vi "sensor wrapper rob.vi"(6 "Degrees":dbl, 8 "error in (no error)":errorcluster, 9 "sensor y":fxp<+/-,64,32>, 10 "Sensor x":fxp<+/-,64,32>, 11 "map reference in":refnum<data-value>) -> (0 "error out":errorcluster, 3 "map reference out 2":refnum<data-value>)   [LabVIEW 2012]
uses:
  <vilib>/rvi/interface/nirviOpenFPGA/nirviOpenFPGA.xnode
  <vilib>/rvi/interface/nirviCloseFPGA/nirviCloseFPGA.xnode
  <vilib>/FPGAPlugInAG/Dynamic/niLvFpga_Close_Dynamic.vi
  <vilib>/rvi/interface/nirviReadWriteControl/nirviReadWriteControl.xnode
  NiFpgaLv.dll
  <vilib>/Utility/error.llb/Error Cluster From Error Code.vi
  <vilib>/rvi/interface/Simulation/niFpgaSimulationCallBeginRW.vi
  <vilib>/rvi/errors/niLvFpgaAdjustHostInterfaceError.vi
  <vilib>/robotics/Navigation/shared/WorldMap/OccupancyGridWorldMap/NI_Robotics_OccupancyGridWorldMap.lvclass
  fpgatrig.vi
  <vilib>/rvi/interface/RandomDataEmulation/nirviRandomDataOpen.vi
  <vilib>/rvi/interface/common/niFpgaCacheSessionInfoDynamic.vi
panel:
  in  "distance":fxp<+/-,64,32>
  out "Rounded y":fxp<+/-,64,32>
  out "Rounded x":fxp<+/-,64,32>
  out "Detected x":fxp<+/-,64,32>
  out "Detected y":fxp<+/-,64,32>
  # "Add into own loop so it updates map independent of disicion making"
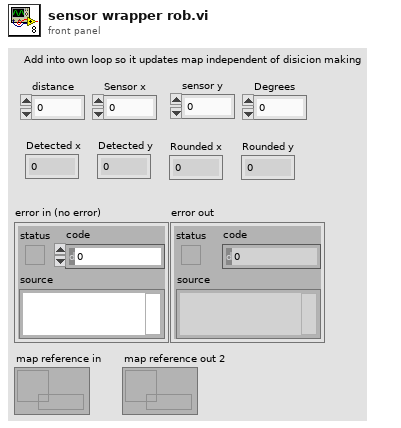
[diagram p1: front panel]
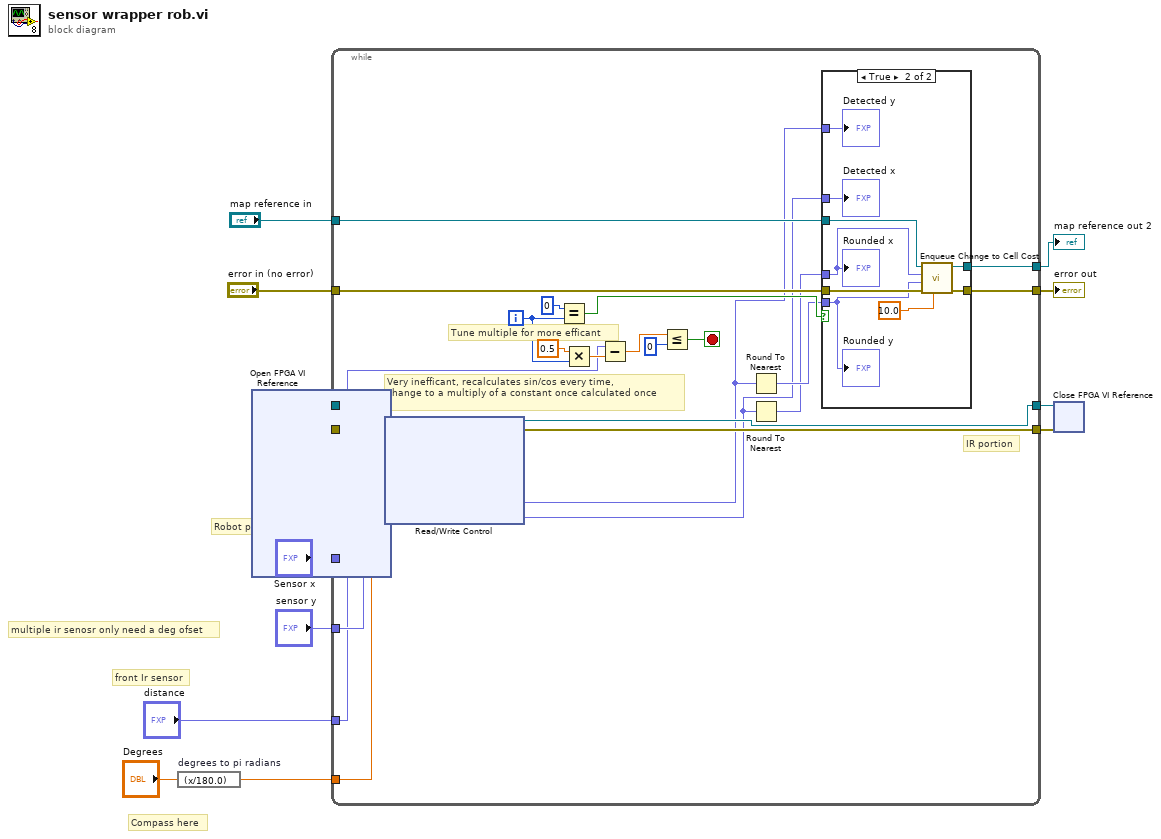
[diagram p0: block diagram]
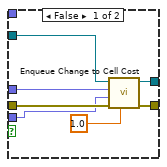
[diagram p2: hidden frame]
diagram:
  # "multiple ir senosr only need a deg ofset"
  # "Robot position"
  # "front Ir sensor"
  # "Compass here"
  n1 = expression code="(x/180.0)" "degrees to pi radians"("Degrees") -> (w9:dbl)
  n2 = xnode "Open FPGA VI Reference"() -> ("FPGA VI Reference Out"=w7:refnum<k20>, "error out"=w8:errorcluster)  [unwired: 2 in]
  n3 = while {
    tunnel: "map reference in" -> [w37]
    tunnel: "error in (no error)" -> [w36]
    tunnel: [w35] -> w4
    tunnel: [w34] -> w3
    tunnel: "sensor y" -> [w16]
    tunnel: "Sensor x" -> [w15]
    tunnel: w9 -> [w18]
    tunnel: "distance" -> [w14]
    tunnel: w8 -> [w24]
    tunnel: w7 -> [w23]
    tunnel: [w22] -> w2
    tunnel: [w21] -> w1
    i -> [w29]
    stop <- w25 stop-if-true
    # "Tune multiple for more efficant"
    # "IR portion"
    # "Very inefficant, recalculates sin/cos every time, \nchange to a multiply of a constant once calculated once"
    n4 = xnode "Read/Write Control"("FPGA VI Reference In"=w23, "error in"=w24, "Sensor position x"=w15, "Sensor position y"=w16, "Distance detected"=w14, "sensor angle (Radiens)"=w18) -> ("FPGA VI Reference Out"=w22:refnum<k20>, "error out"=w21:errorcluster, "Detected y Cord"=w20:fxp<+/-,64,32>, "Detected x Cord"=w19:fxp<+/-,64,32>)
    n5 = Equal?(x=0, y=w29) -> (x = y?=w32:bool)
    n6 = Multiply(x=0.5, y=w29) -> (x*y=w27:dbl)
    n7 = Subtract(x=w14, y=w27) -> (x-y=w17:dbl)
    n8 = Less Or Equal?(x=w17, y=0) -> (x <= y?=w25:bool)
    n9 = Round To Nearest(number=w20) -> (nearest integer value=w31:fxp<+/-,33,33>)
    n10 = Round To Nearest(number=w19) -> (nearest integer value=w30:fxp<+/-,33,33>)
    n11 = case shown="True" w32 {
      tunnel: w37 -> [w40 w53]
      tunnel: w36 -> [w41 w52]
      tunnel: [w43 w50] -> w35
      tunnel: [w42 w49] -> w34
      tunnel: w30 -> [w39 w45]
      tunnel: w31 -> [w38 w46]
      tunnel: w19 -> [_ w48]
      tunnel: w20 -> [_ w47]
      frame False {
        n12 = call <vilib>:"Enqueue Change to Cell Cost.vi"("cost"=1.0, "error in (no error)"=w41, "y"=w38, "x"=w39, "map reference in"=w40) -> ("error out"=w42:errorcluster, "map reference out"=w43:refnum<data-value>)  [unwired: 5 in]
      }
      frame True {
        n13 = call <vilib>:"Enqueue Change to Cell Cost.vi"("cost"=10.0, "error in (no error)"=w52, "y"=w46, "x"=w45, "map reference in"=w53) -> ("error out"=w49:errorcluster, "map reference out"=w50:refnum<data-value>)  [unwired: 5 in]
        "Rounded y" <- w46
        "Rounded x" <- w45
        "Detected x" <- w48
        "Detected y" <- w47
      }
    }
  }
  "map reference out 2" <- w4
  "error out" <- w3
  n14 = xnode "Close FPGA VI Reference"("FPGA VI Reference In"=w2, "error in"=w1) -> ()  [unwired: 1 out]
